vi "JoystickRateLimiter.vi"(4 "Vertical (Y) Multiplier":dbl=0.7, 6 "Horizontal (X) Multiplier":dbl=0.45, 7 "output rate (Joystick Percentage/Second)":dbl=140.0 format="%.2f", 8 "Direction Toggle":bool, 9 "Y Input":dbl, 10 "X Input":dbl, 11 "Bypass":bool) -> (1 "Left Motor Value":dbl, 2 "Right Motor Value":dbl)   [LabVIEW 2019]
uses:
  <vilib>/addons/control/pid/pid.llb/PID Output Rate Limiter (DBL).vi
  <vilib>/Rock Robotics/WPI/Joystick/WPI_JoystickArcadeMapping.vi
  <vilib>/addons/control/pid/NI_PID_pid.lvlib
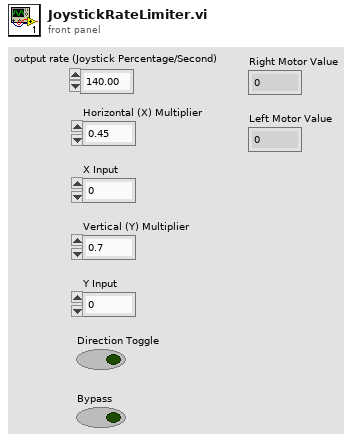
[diagram p1: front panel]
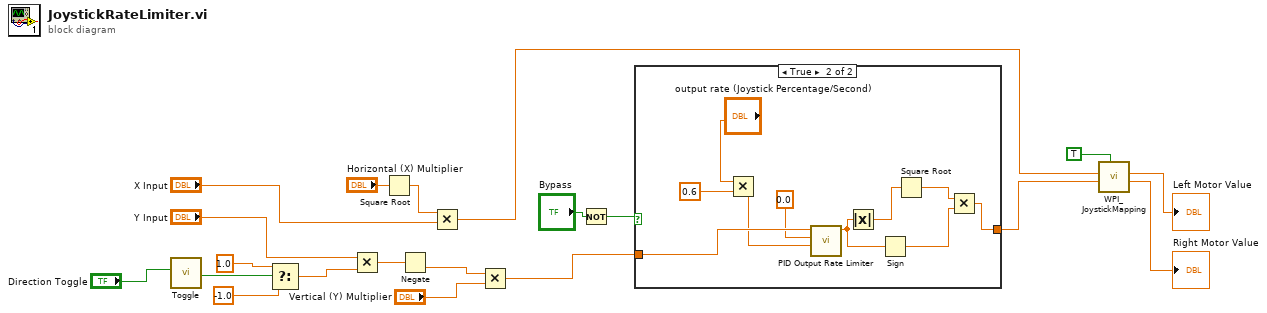
[diagram p0: block diagram]
diagram:
  n1 = call "Toggle.vi"("Input"="Direction Toggle") -> ("Output"=w11:bool)  [unwired: 10 in]
  n2 = Select(t=1.0, s=w11, f=-1.0) -> (s? t:f=w12:dbl)
  n3 = Multiply(x="Y Input", y=w12) -> (x*y=w9:dbl)
  n4 = Square Root(x="Horizontal (X) Multiplier") -> (sqrt(x)=w18:dbl)
  n5 = Negate(x=w9) -> (-x=w15:dbl)
  n6 = Multiply(x="X Input", y=w18) -> (x*y=w20:dbl)
  n7 = Multiply(x=w15, y="Vertical (Y) Multiplier") -> (x*y=w16:dbl)
  n8 = Not(x="Bypass") -> (.not. x?=w1:bool)
  n9 = case shown="True" w1 {
    tunnel: w16 -> [w21 w31]
    tunnel: [w21 w25] -> w17
    frame False {
    }
    frame True {
      n10 = Multiply(x="output rate (Joystick Percentage/Second)", y=0.6) -> (x*y=w28:dbl)
      n11 = call-poly <vilib>:"PID Output Rate Limiter.vi"("output rate (EGU/min)"=w28, "initial output"=0.0, "input (controller output)"=w31) -> ("output"=w23:dbl)  [unwired: 5 in, 1 out]
      n12 = Absolute Value(x=w23) -> (abs(x)=w24:dbl)
      n13 = Sign(1:w23) -> (0:w22:dbl)
      n14 = Square Root(x=w24) -> (sqrt(x)=w26:dbl)
      n15 = Multiply(x=w26, y=w22) -> (x*y=w25:dbl)
    }
  }
  n16 = call-poly <vilib>:"WPI_JoystickMapping.vi"("Square Inputs"=TRUE, "Y axis value"=w17, "X axis value"=w20) -> ("Right Motor Value"=→"Right Motor Value":dbl, "Left Motor Value"=→"Left Motor Value":dbl)  [unwired: 7 in]
